vi "Read LNA.vi"(11 "CS++RTMainActor in":refnum<class "CS++RTMainActor.lvclass">) -> (2 "Actor Framework:Message Enqueuer":refnum<class "Message Enqueuer.lvclass">, 3 "CS++RTMainActor out":refnum<class "CS++RTMainActor.lvclass">)   [LabVIEW 2015, in "CS++RTMain.lvlib" / "CS++RTMainActor.lvclass"]
uses:
  CS++RTMainActor.lvclass
  <vilib>/ActorFramework/Message Enqueuer/Message Enqueuer.lvclass
  CS++RTMainActor.lvclass/CS++RTMainActor.ctl
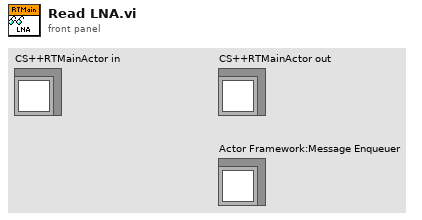
[diagram p1: front panel]
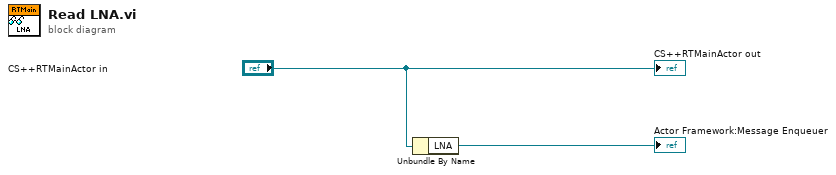
[diagram p0: block diagram]
diagram:
  n1 = Unbundle By Name("CS++RTMainActor in") -> ("LNA"=→"Actor Framework:Message Enqueuer":refnum<class "Message Enqueuer.lvclass">)
  "CS++RTMainActor out" <- "CS++RTMainActor in"
